vi "Teleop.vi"(10 "Match Info":T1={"Autonomous Elapsed Seconds"=0.0, "TeleOp Elapsed Seconds"=0.0, "Disabled Elapsed Seconds"=0.0, "Visited Autonomous"=FALSE, "Visited TeleOp"=FALSE, "Visited Disabled"=FALSE, "Autonomous Settings"={"Autonomous Style"=enum."Independent", "VI Refnum"=refnum}}, 11 "Call Context":T2) -> ()   [LabVIEW 2014]
doc: "This VI is called for each TeleOp packet received from the DS where the robot is not disabled. It is often used to read from the joysticks and update I/O or to update setpoints for timed control loops. It should complete and return within 20 milliseconds or it may miss DS packets."
uses:
  <vilib>/Rock Robotics/WPI/DriverStation/WPI_DriverStationDerivedRobotMode.ctl
  <vilib>/Rock Robotics/WPI/DriverStation/WPI_DriverStationMatch Info.ctl
  <vilib>/Rock Robotics/WPI/RobotDrive/WPI_RobotDriveGetSetRefNum.vi
  <vilib>/Rock Robotics/WPI/Joystick/WPI_JoystickGetSetRefNum.vi
  <vilib>/Rock Robotics/Network Tables/SD Write Boolean Array.vi
  <vilib>/Rock Robotics/Network Tables/SD Write Numeric Array.vi
  <vilib>/Rock Robotics/Network Tables/SD Read Boolean.vi
  <vilib>/Rock Robotics/Network Tables/SD Read Number.vi
panel:
  out "Sample Slider 0":dbl(slide) scale=0.0..5.0
  out "Sample Boolean 1":bool
  out "Sample Boolean 0":bool
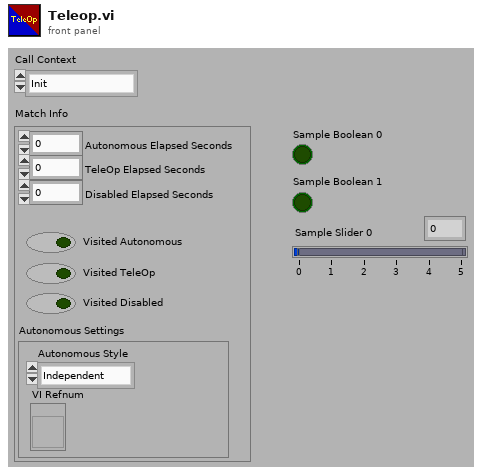
[diagram p1: front panel]
types:
  T1 = typedef "WPI_DriverStationMatch Info.ctl" = cluster{"Autonomous Elapsed Seconds":dbl, "TeleOp Elapsed Seconds":dbl, "Disabled Elapsed Seconds":dbl, "Visited Autonomous":bool, "Visited TeleOp":bool, "Visited Disabled":bool, "Autonomous Settings":cluster{"Autonomous Style":enum16{"Iterative", "Independent"}, "VI Refnum":refnum<vi>}}
  T2 = typedef "WPI_DriverStationDerivedRobotMode.ctl" = enum16{"Init", "Execute", "Stop"}
  T3 = typedef "WPI_RobotDriveDevRef.ctl" = cluster{"DevStatus":errorcluster, "Motors[]":T4[], "Square Inputs":bool, "Max Output":dbl}
  T4 = typedef "WPI_MotorControlDeviceRef.ctl" = cluster{"DeviceStatus":errorcluster, "Type":T5, "PWM":cluster{"Controller":T6, "PWM Channel":T7, "DeadBand":T8}, "CAN":cluster{"Device Number":u8, "Control Mode":T9, "Semaphore":T10, "Max Vout":dbl, "TalonSRX Control Mode":T11}, "Invert":bool, "TransformRef":T12, "InvTransformRef":T12}
  T5 = typedef "WPI_MotorControlType.ctl" = enum16{"PWM", "CAN", "CANTalonSRX"}
  T6 = typedef "FPGA_TypedefDigitalModule.ctl" = enum16{"Controller 1"}
  T7 = typedef "FPGA_DIOPWMChannel.ctl" = enum8{"PWM 0", "PWM 1", "PWM 2", "PWM 3", "PWM 4", "PWM 5", "PWM 6", "PWM 7", "PWM 8", "PWM 9", "PWM MXP 0", "PWM MXP 1", "PWM MXP 2", "PWM MXP 3", "PWM MXP 4", "PWM MXP 5", "PWM MXP 6", "PWM MXP 7", "PWM MXP 8", "PWM MXP 9", "Invalid"}
  T8 = typedef "WPI_PWMDeadband.ctl" = cluster{"Name":string, "maxPositivePwm":i32, "minPositivePwm":i32, "centerPwm":i32, "maxNegativePwm":i32, "minNegativePwm":i32, "angularRange":u16}
  T9 = typedef "WPI_CANJaguar_ControlMode.ctl" = enum8{"Percent VBus", "Current", "Speed", "Position", "Voltage"}
  T10 = typedef "Semaphore RefNum" = refnum<k1>
  T11 = typedef "WPI_CANTalonSRX_APIControlMode.ctl" = enum8{"Percent VBus", "Speed", "Position", "Slave", "Unchanged / Invalid"}
  T12 = typedef "WPI_PWMTransform_ConPane.ctl" = refnum<vi>
  T13 = typedef "WPI_JoystickDevRef.ctl" = cluster{"Device":T14}
  T14 = typedef "WPI_JoystickDeviceEnum.ctl" = enum16{"USB 0", "USB 1", "USB 2", "USB 3", "USB 4", "USB 5"}
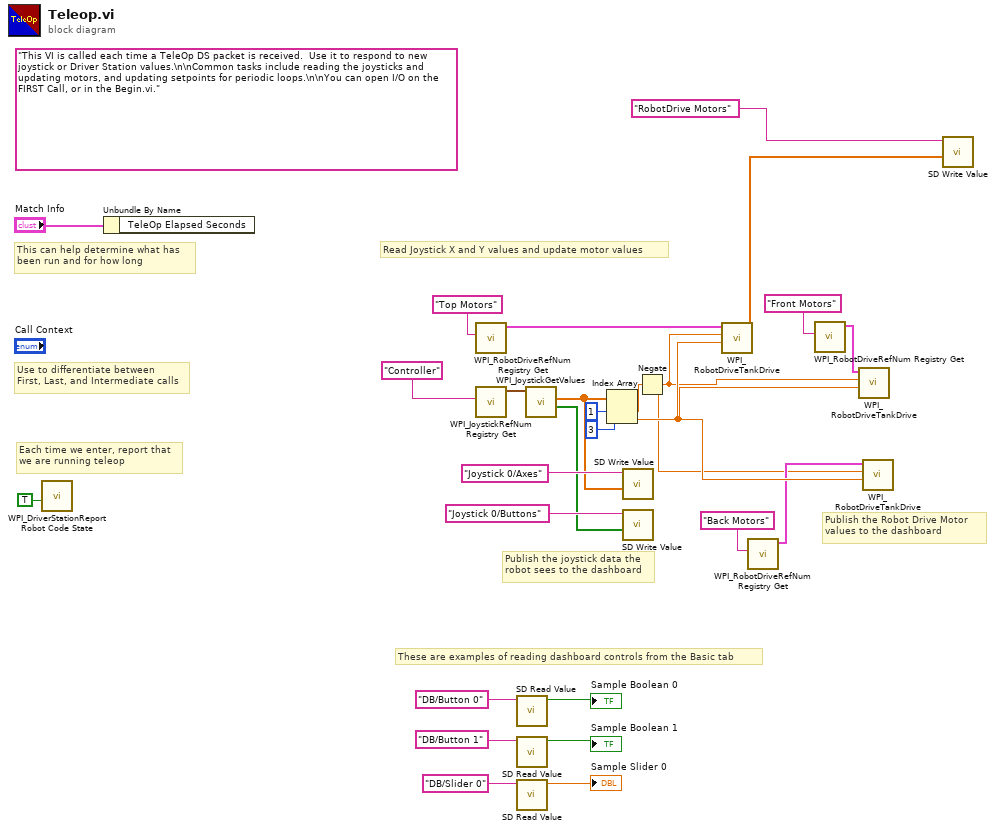
[diagram p0: block diagram]
diagram:
  (unwired) "This VI is called each time a TeleOp DS packet is received.  Use it to respond to new joystick or Driver Station values.\n\nCommon tasks include reading the joysticks and updating motors, and updating setpoints for periodic loops.\n\nYou can open I/O on the FIRST Call, or in the Begin.vi."
  # "These are examples of reading dashboard controls from the Basic tab"
  # "Publish the Robot Drive Motor\nvalues to the dashboard"
  # "Publish the joystick data the\nrobot sees to the dashboard"
  # "Each time we enter, report that\nwe are running teleop"
  # "Use to differentiate between\nFirst, Last, and Intermediate calls"
  # "This can help determine what has\nbeen run and for how long"
  # "Read Joystick X and Y values and update motor values"
  n1 = call <vilib>:"WPI_DriverStationReport Robot Code State.vi"("TeleOp"=TRUE ("Autonomous")) -> ()  [unwired: 10 in, 1 out]
  n2 = Unbundle By Name("Match Info") -> ()  [unwired: 1 out]
  n3 = call <vilib>:"WPI_RobotDriveRefNum Registry Get.vi"("refnum name"="Top Motors") -> ("RobotDriveDevRef"=w25:T3)  [unwired: 1 in, 9 out]
  n4 = call <vilib>:"WPI_JoystickRefNum Registry Get.vi"("refnum name"="Controller") -> ("JoystickDevRef"=w23:T13)  [unwired: 1 in, 9 out]
  n5 = call-poly <vilib>:"SD Read Value.vi"("Name"="DB/Button 0" ("refnum name")) -> ("Boolean"=→"Sample Boolean 0":bool)  [unwired: 8 in, 2 out]
  n6 = call-poly <vilib>:"SD Read Value.vi"("Name"="DB/Button 1" ("refnum name")) -> ("Boolean"=→"Sample Boolean 1":bool)  [unwired: 8 in, 2 out]
  n7 = call-poly <vilib>:"SD Read Value.vi"("Name"="DB/Slider 0" ("refnum name")) -> ("Numeric"=→"Sample Slider 0":dbl)  [unwired: 8 in, 2 out]
  n8 = call <vilib>:"WPI_JoystickGetValues.vi"("JoystickDevRef"=w23) -> ("Buttons"=w10:bool[], "Axes"=w12:dbl[])  [unwired: 6 in, 3 out]
  n9 = Index Array(array=w12, index #1=1 ("index"), index #2=3 ("index")) -> (element #1=w9:dbl, element #2=w8:dbl)
  n10 = call-poly <vilib>:"SD Write Value.vi"("Numeric Array"=w12, "Name"="Joystick 0/Axes") -> ()  [unwired: 8 in, 2 out]
  n11 = call-poly <vilib>:"SD Write Value.vi"("Boolean Array"=w10, "Name"="Joystick 0/Buttons") -> ()  [unwired: 8 in, 2 out]
  n12 = Negate(x=w9) -> (-x=w1:dbl)
  n13 = call <vilib>:"WPI_RobotDriveTankDrive.vi"("Right axis value"=w8, "Left axis value"=w1, "RobotDriveDevRef"=w25) -> ("Motor Values"=w14:dbl[])  [unwired: 6 in, 2 out]
  n14 = call <vilib>:"WPI_RobotDriveRefNum Registry Get.vi"("refnum name"="Back Motors") -> ("RobotDriveDevRef"=w4:T3)  [unwired: 1 in, 9 out]
  n15 = call <vilib>:"WPI_RobotDriveRefNum Registry Get.vi"("refnum name"="Front Motors") -> ("RobotDriveDevRef"=w5:T3)  [unwired: 1 in, 9 out]
  n16 = call <vilib>:"WPI_RobotDriveTankDrive.vi"("Right axis value"=w8, "Left axis value"=w1, "RobotDriveDevRef"=w5) -> ()  [unwired: 6 in, 3 out]
  n17 = call <vilib>:"WPI_RobotDriveTankDrive.vi"("Right axis value"=w8, "Left axis value"=w1, "RobotDriveDevRef"=w4) -> ()  [unwired: 6 in, 3 out]
  n18 = call-poly <vilib>:"SD Write Value.vi"("Numeric Array"=w14, "Name"="RobotDrive Motors") -> ()  [unwired: 8 in, 2 out]
